vi "LEDMATRIX.vi"() -> ()   [LabVIEW 2015]
uses:
  Controls/HID Data.ctl
  <vilib>/userdefined/High Color/IMAQdx.ctl
  <vilib>/vision/Image Controls.llb/IMAQ Image.ctl
  Controls/HID State.ctl
  Controls/FGV_Options.ctl
panel:
  out "TXT_003":string
  in  "LBL_015":u16(ring)=3 caption="Cor de Fundo" items=["Verde", "Azul", "Vermelho", "Branco", "Rosa", "Amarelo", "Turquesa", "Preto"]
  in  "LBL_014":u16(ring)=2 caption="Cor Frontal" items=["Verde", "Azul", "Vermelho", "Branco", "Rosa", "Amarelo", "Turquesa", "Preto"]
  in  "BOOL_004":bool
  in  "BOOL_003":bool
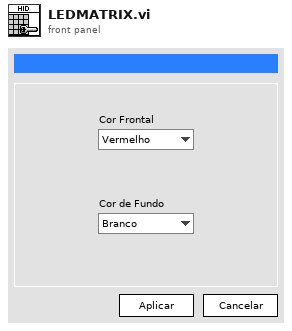
[diagram p1: front panel]
types:
  T1 = typedef "FGV_Options.ctl" = enum16{"Read from File", "Write to File", "Get", "Set"}
  T2 = typedef "HID Data.ctl" = cluster{"IMAQdx Session":T3, "Resampled Image":T4, "Low Level Grab":T4, "X Resolution":i32, "Y Resolution":i32, "Image Threshold":u8, "Reset Value":i32, "FIFO Timer":u16, "Row Timer":u32, "Memory Writer Timer":u8, "Color":enum16{"Green", "Blue", "Red", "White", "Pink", "Yellow", "Turquoise", "Black"}, "Top":bool[][], "Bottom":bool[][], "Timeout (ms)":i32, "Menu Tag":string, "Color Background":enum16{"Green", "Blue", "Red", "White", "Pink", "Yellow", "Turquoise", "Black"}, "FPGA VI Reference":refnum<k20>, "Next Steps":T5[], "Turn off LED Matrix":bool, "FPGA Alias":string, "FPGA Bitfile":path, "Localized Texts":cluster{"Status Text":cluster{"Status Text Table":string[], "Status Text Index":i32}, "Controls":cluster{"Control Text Table":string[], "Control Text Index":i32}, "Titles":cluster{"Titles Text Table":string[], "Titles Text Index":i32}}, "Language":u16}
  T3 = typedef "IMAQdx.ctl" = refnum<k21>
  T4 = typedef "IMAQ Image.ctl" = refnum<image>
  T5 = typedef "HID State.ctl" = enum16{"Initialize", "Set FPGA Parametes", "Set Camera Parameters", "Set LED Matrix Parameters", "Initialize FPGA Interface", "Initialize Camera", "Start FPGA VI", "Start Camera", "Wait for Event", "Update UI", "Acquire", "Process Image", "Get Boolean Arrays", "Send to FPGA", "Menu Pop-Up", "Menu Actions", "Handle Errors", "Close Camera", "Close FPGA", "Stop", "Exit"}
  T6 = enum16{"Green", "Blue", "Red", "White", "Pink", "Yellow", "Turquoise", "Black"}
  T7 = enum16{"Green", "Blue", "Red", "White", "Pink", "Yellow", "Turquoise", "Black"}[]
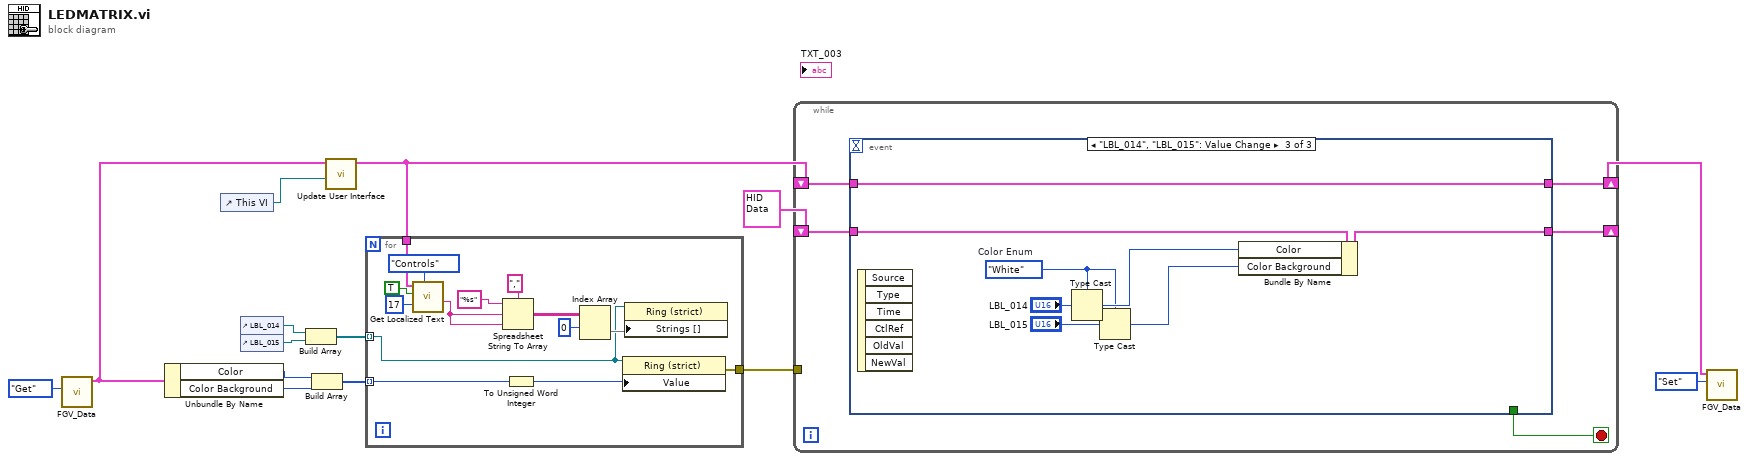
[diagram p0: block diagram]
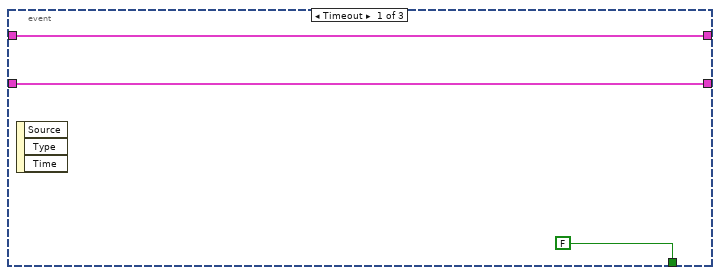
[diagram p2: hidden frame]
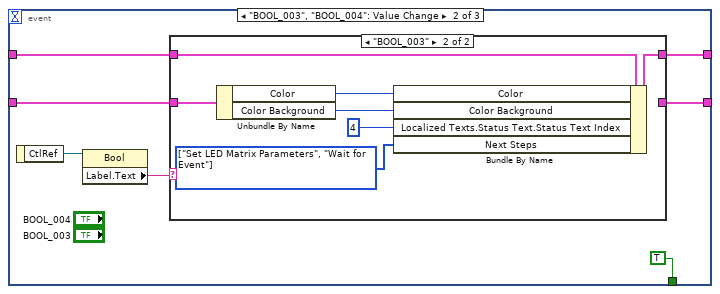
[diagram p3: hidden frame]
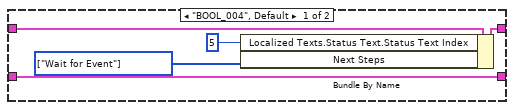
[diagram p4: hidden frame]
diagram:
  n1 = call "FGV_Data.vi"("Option"=FGV_Options."Get") -> ("Data Out"=w5:T2)  [unwired: 9 in, 1 out]
  n2 = Unbundle By Name(w5) -> ("Color"=w11:T6, "Color Background"=w12:T6)
  n3 = control-ref of="This VI"() -> (w2:refnum<vi>)
  n4 = control-ref of="LBL_014"() -> (w8:refnum<vi>)
  n5 = control-ref of="LBL_015"() -> (w9:refnum<vi>)
  n6 = Build Array(w8, w9) -> (w10:refnum<vi>[])
  n7 = Build Array(w11, w12) -> (w13:T7)
  n8 = call "Update User Interface.vi"("VI Refnum"=w2, "Data In"=w5) -> ("Data Out"=w1:T2)  [unwired: 8 in, 1 out]
  n9 = for {
    tunnel: w10 -> [w17] mode=indexing
    tunnel: w13 -> [w28] mode=indexing
    tunnel: [w27] -> w7
    tunnel: w1 -> [w26]
    n10 = call "Get Localized Text.vi"("Text Type"=enum16{"Status", "Title", "Controls"}."Controls", "Text Index"=17, "Force Index"=TRUE, "Data In"=w26) -> ("Localized Text"=w18:string)  [unwired: 6 in, 1 out]
    n11 = Spreadsheet String To Array(delimiter (Tab)=",", format string="%s", spreadsheet string=w18, array type (2D Dbl)=w18) -> (array=w21:string[][])
    n12 = To Unsigned Word Integer(number=w28) -> (unsigned 16bit integer=w15:u16)
    n13 = Index Array(array=w21, index (row)=0) -> (element=w19:string[])  [unwired: 1 in]
    n14 = property class="Ring (strict)"(reference=w17, "Value"=w15) -> (error out=w27:errorcluster)  [unwired: 1 in, 1 out]
    n15 = property class="Ring (strict)"(reference=w17, "Strings []"=w19) -> ()  [unwired: 1 in, 2 out]
  }
  n16 = while {
    shift-right: [w33] -> w3
    shift-left: w1 -> [w32]
    shift-right: [w29] -> _
    shift-left: T2 {"IMAQdx Session"="", "Resampled Image"=refnum, "Low Level Grab"=refnum, "X Resolution"=0, "Y Resolution"=0, "Image Threshold"=0, "Reset Value"=0, "FIFO Timer"=0, "Row Timer"=0, "Memory Writer Timer"=0, "Color"=enum."Red", "Top"=array32x96[3072 elements], "Bottom"=array32x96[3072 elements], "Timeout (ms)"=0, "Menu Tag"="", "Color Background"=enum."White", "FPGA VI Reference"=refnum, "Next Steps"=[], "Turn off LED Matrix"=FALSE, "FPGA Alias"="", "FPGA Bitfile"=path "", "Localized Texts"={"Status Text"={"Status Text Table"=[], "Status Text Index"=0}, "Controls"={"Control Text Table"=[], "Control Text Index"=0}, "Titles"={"Titles Text Table"=[], "Titles Text Index"=0}}, "Language"=0} ("Data In TMP") -> [w30]
    tunnel: w7 -> [_]
    stop <- w31 stop-if-true
    n17 = event shown="[2] \"LBL_014\", \"LBL_015\": Value Change" {
      selector: _ -> [_ _ _]
      dyn-events: _ -> [_ _ _]
      timeout: _ -> [_ _ _]
      tunnel: [w36 w40 w63] -> w33
      tunnel: w32 -> [w36 w41 w63]
      tunnel: [FALSE TRUE _] -> w31
      tunnel: w30 -> [w34 w38 w59]
      tunnel: [w34 w37 w62] -> w29
      event Timeout {
        n18 = event-data() -> ()  [unwired: 1 in, 3 out]
      }
      event "BOOL_003", "BOOL_004": Value Change {
        n19 = event-data() -> ("CtlRef"=w42:refnum<vi>)  [unwired: 1 in]
        n20 = property class="Bool"(reference=w42) -> ("Label.Text"=w39:string)  [unwired: 1 in, 2 out]
        n21 = case shown="\"BOOL_003\"" w39 {
          tunnel: w41 -> [w48 w55]
          tunnel: [w46 w54] -> w40
          tunnel: w38 -> [w47 w53]
          tunnel: [w47 _] -> w37
          frame "BOOL_004", Default {
            w45 = T5[] [enum."Wait for Event"] items=["Initialize", "Set FPGA Parametes", "Set Camera Parameters", "Set LED Matrix Parameters", "Initialize FPGA Interface", "Initialize Camera", "Start FPGA VI", "Start Camera", "Wait for Event", "Update UI", "Acquire", "Process Image", "Get Boolean Arrays", "Send to FPGA", "Menu Pop-Up", "Menu Actions", "Handle Errors", "Close Camera", "Close FPGA", "Stop", "Exit"] ("Array")
            n22 = Bundle By Name(cluster=w48, "Localized Texts.Status Text.Status Text Index"=5 ("Status"), "Next Steps"=w45) -> (w46:T2)
          }
          frame "BOOL_003" {
            w50 = T5[] [enum."Set LED Matrix Parameters", enum."Wait for Event"] items=["Initialize", "Set FPGA Parametes", "Set Camera Parameters", "Set LED Matrix Parameters", "Initialize FPGA Interface", "Initialize Camera", "Start FPGA VI", "Start Camera", "Wait for Event", "Update UI", "Acquire", "Process Image", "Get Boolean Arrays", "Send to FPGA", "Menu Pop-Up", "Menu Actions", "Handle Errors", "Close Camera", "Close FPGA", "Stop", "Exit"] ("Array")
            n23 = Unbundle By Name(w53) -> ("Color"=w52:T6, "Color Background"=w51:T6)
            n24 = Bundle By Name(cluster=w55, "Color"=w52, "Color Background"=w51, "Localized Texts.Status Text.Status Text Index"=4 ("Status"), "Next Steps"=w50) -> (w54:T2)
          }
        }
      }
      event "LBL_014", "LBL_015": Value Change {
        w56 = T6."White"  # Color Enum
        n25 = event-data() -> ()  [unwired: 1 in, 6 out]
        n26 = Type Cast(type=w56, x="LBL_014") -> (*(type *) &x=w58:T6)
        n27 = Type Cast(type=w56, x="LBL_015") -> (*(type *) &x=w57:T6)
        n28 = Bundle By Name(cluster=w59, "Color"=w58, "Color Background"=w57) -> (w62:T2)
      }
    }
  }
  n29 = call "FGV_Data.vi"("Option"=FGV_Options."Set", "Data In"=w3) -> ()  [unwired: 8 in, 2 out]
